vi "Write connection ID.vi"(5 "connection ID":refnum<k5>, 9 "Downloader in":refnum<class "Downloader.lvclass">) -> (3 "Downloader out":refnum<class "Downloader.lvclass">)   [LabVIEW 2014, in "Raspberry Pi Compatible Compiler for LabVIEW.lvlib" / "Downloader.lvclass"]
uses:
  Downloader.lvclass
  Downloader.lvclass/Downloader.ctl
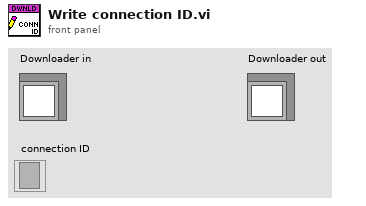
[diagram p1: front panel]
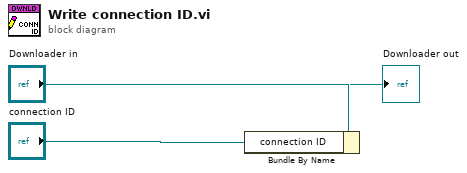
[diagram p0: block diagram]
diagram:
  n1 = Bundle By Name(cluster="Downloader in", "connection ID"="connection ID") -> (→"Downloader out":refnum<class "Downloader.lvclass">)
